vi "Device Property - Set Timeout.vi"(8 "error in (no error)":errorcluster, 10 "Timout":i32, 11 "Device Ref in":T1 format="%.0x") -> (0 "error out":errorcluster, 3 "Device Ref out":T1 format="%.0x")   [LabVIEW 2017]
doc: "Gets the IP Address of the custom device target."
uses:
  <vilib>/NI Veristand/Custom Device API/Custom Device Item Ref.ctl
  SV Global.vi
  <vilib>/NI Veristand/Custom Device API/Set Item Property (I32).vi
  <vilib>/NI Veristand/Custom Device API/Custom Device API.lvlib
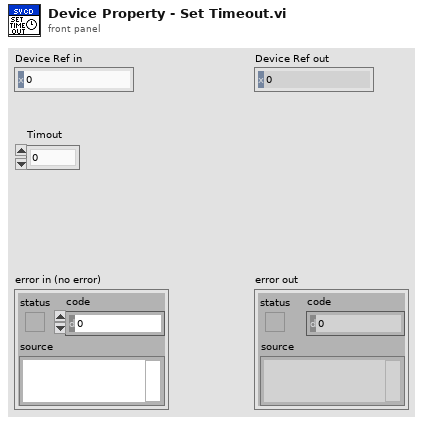
[diagram p1: front panel]
types:
  T1 = typedef "Custom Device API.lvlib/Custom Device Item Ref.ctl" = u64
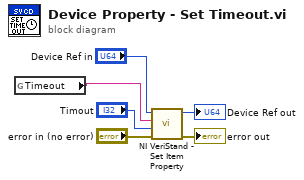
[diagram p0: block diagram]
diagram:
  n1 = global read "SV Global.vi" "Timeout"() -> (w1:string)
  n2 = call-poly <vilib>:"NI VeriStand - Set Item Property.vi"("error in (no error)"="error in (no error)", "Value"="Timout", "Property Name"=w1, "Item Ref in"="Device Ref in") -> ("error out"=→"error out":errorcluster, "Item Ref out"=→"Device Ref out":T1)  [unwired: 5 in, 1 out]
